vi "Log_MessageHandler_WriteMessageIntoLogFile.vi"(8 "error in (no error)":errorcluster, 10 "Messages.lvclass":refnum<class "Messages.lvclass">, 11 "MessageHandler in":refnum<class "MessageHandler.lvclass">) -> (0 "error out":errorcluster, 3 "MessageHandler out":refnum<class "MessageHandler.lvclass">)   [LabVIEW 2013, in "MessageHandler.lvclass"]
uses:
  MessageHandler.lvclass
  001 - MAIN/Class/Messages/Messages.lvclass
  030 - EVENTS/03 - ToMessageHandlerProcess/ToMessageHandlerEvent.ctl
  030 - EVENTS/03 - ToMessageHandlerProcess/enumMessageCriticity.ctl
  MessageHandler.lvclass/MessageHandler.ctl
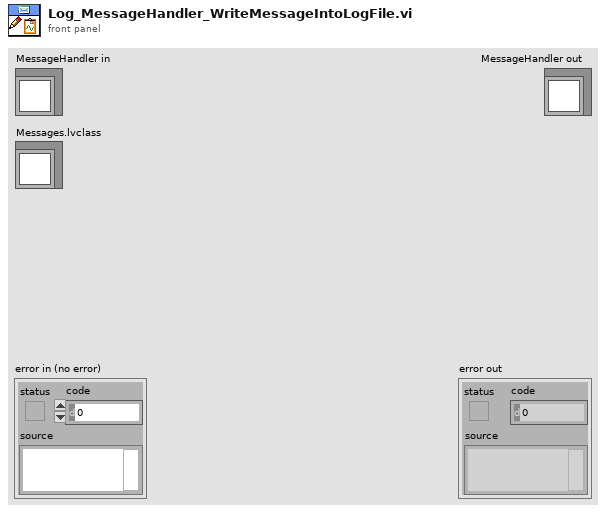
[diagram p1: front panel]
types:
  T1 = typedef "ToMessageHandlerEvent.ctl" = cluster{"date / time":timestamp, "Criticity":T2, "Emitter":string, "Message":string}
  T2 = typedef "enumMessageCriticity.ctl" = enum16{"No error", "Info", "Warning", "Error", "Fatal error"}
  T3 = enum16{"open", "replace", "create", "open or create", "replace or create", "replace or create with confirmation"}
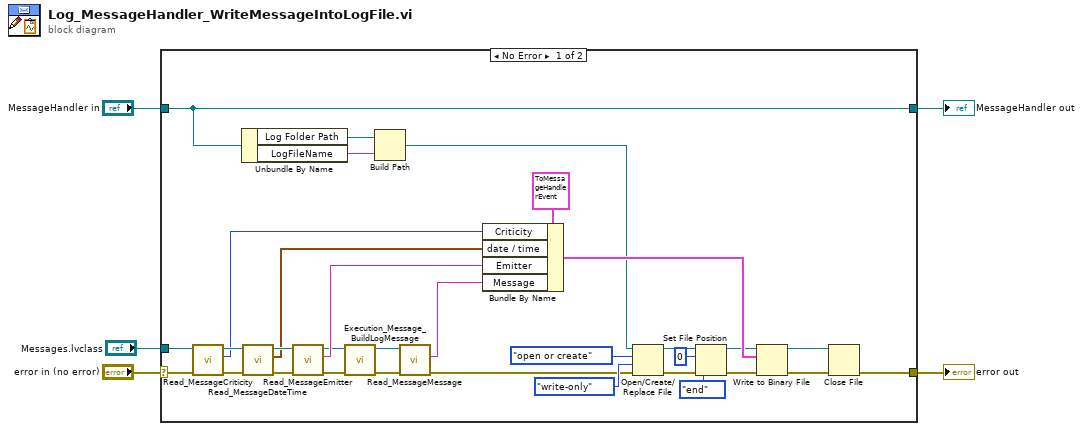
[diagram p0: block diagram]
diagram:
  n1 = case shown="No Error" "error in (no error)" {
    selector: "error in (no error)" -> [w32 w39]
    tunnel: [w20 w39] -> w4
    tunnel: [w19 w38] -> w2
    tunnel: "MessageHandler in" -> [w19 w38]
    tunnel: "Messages.lvclass" -> [w31 _]
    frame No Error {
      n2 = call-dynamic "Read_MessageCriticity.vi"("error in (no error)"=w32, "Messages in"=w31) -> ("error out"=w34:errorcluster, "Criticity"=w14:T2, "Messages out"=w36:refnum<class "Messages.lvclass">)  [unwired: 7 in]
      n3 = Unbundle By Name(w19) -> ("Log Folder Path"=w18:path, "LogFileName"=w17:string)
      n4 = call-dynamic "Read_MessageDateTime.vi"("error in (no error)"=w34, "Messages in"=w36) -> ("error out"=w33:errorcluster, "date / time"=w13:timestamp, "Messages out"=w35:refnum<class "Messages.lvclass">)  [unwired: 7 in]
      n5 = call-dynamic "Read_MessageEmitter.vi"("error in (no error)"=w33, "Messages in"=w35) -> ("error out"=w10:errorcluster, "Emitter"=w12:string, "Messages out"=w11:refnum<class "Messages.lvclass">)  [unwired: 7 in]
      n6 = call-dynamic "Execution_Message_BuildLogMessage.vi"("error in (no error)"=w10, "Messages in"=w11) -> ("error out"=w9:errorcluster, "Messages out"=w7:refnum<class "Messages.lvclass">)  [unwired: 8 in]
      n7 = Build Path(base path=w18, name or relative path=w17) -> (appended path=w16:path)
      n8 = call-dynamic "Read_MessageMessage.vi"("error in (no error)"=w9, "Messages in"=w7) -> ("error out"=w8:errorcluster, "Message"=w6:string)  [unwired: 7 in, 1 out]
      n9 = Bundle By Name(cluster=T1 {"date / time"=timestamp(0 s since 1904-01-01), "Criticity"=enum."No error", "Emitter"="", "Message"=""} ("Message"), "Criticity"=w14, "date / time"=w13, "Emitter"=w12, "Message"=w6) -> (w37:T1)
      n10 = Open/Create/Replace File(file path (use dialog)=w16, error in=w8, operation (0:open)=T3."open or create", access (0:read/write)=enum16{"read/write", "read-only", "write-only"}."write-only") -> (refnum out=w26:refnum<file>, error out=w24:errorcluster)  [unwired: 2 in, 1 out]
      n11 = Set File Position(offset (in bytes) (0)=i64 0, refnum=w26, from (0:start)=enum16{"start", "end", "current"}."end", error in=w24) -> (refnum out=w25:refnum<file>, error out=w23:errorcluster)
      n12 = Write to Binary File(file (use dialog)=w25, data=w37, error in=w23) -> (refnum out=w27:refnum<file>, error out=w28:errorcluster)  [unwired: 3 in, 1 out]
      n13 = Close File(refnum=w27, error in=w28) -> (error out=w20:errorcluster)  [unwired: 1 out]
    }
    frame Error {
    }
  }
  "error out" <- w4
  "MessageHandler out" <- w2
